vi "SysExe.Test Async StdIn and StdOut.vi"() -> ()   [LabVIEW 2018]
panel:
  in  "App":path=path "cmd.exe"
  out "Error":errorcluster
  out "Write StdIn":errorcluster
  out "StdOut":string
  in  "StdIn":string
  in  "stop":bool
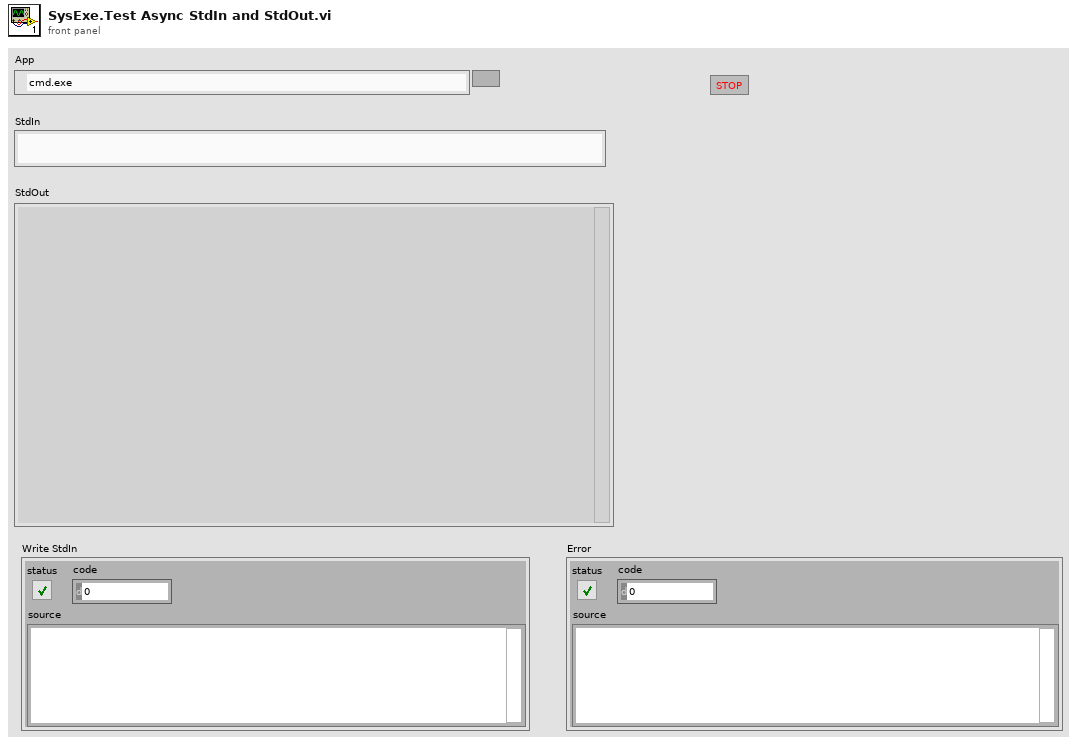
[diagram p1: front panel]
types:
  T1 = cluster{"Process":refnum<k24>, "StdIn":refnum<k24>, "StdErr":refnum<k24>, "StdOut":refnum<k24>, "StdOutDat":string, "StdErrDat":string, "StdInDat":string, "Args":string, "App":string, "AppFolder":path, "WorkingFolder":path, "IsRunning":bool, "Error":errorcluster, "StdOutCallback":refnum<k27>}
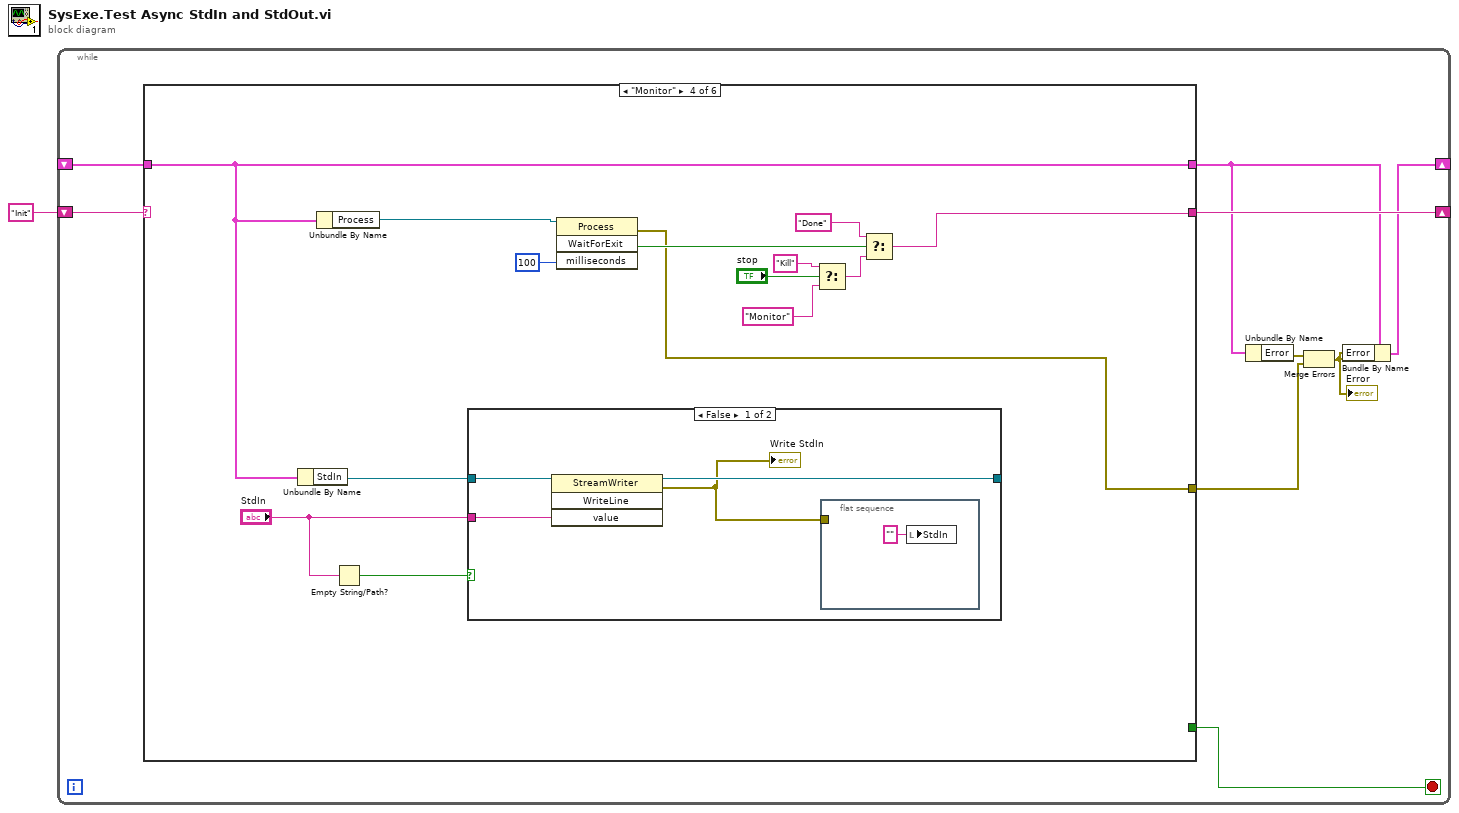
[diagram p0: block diagram]
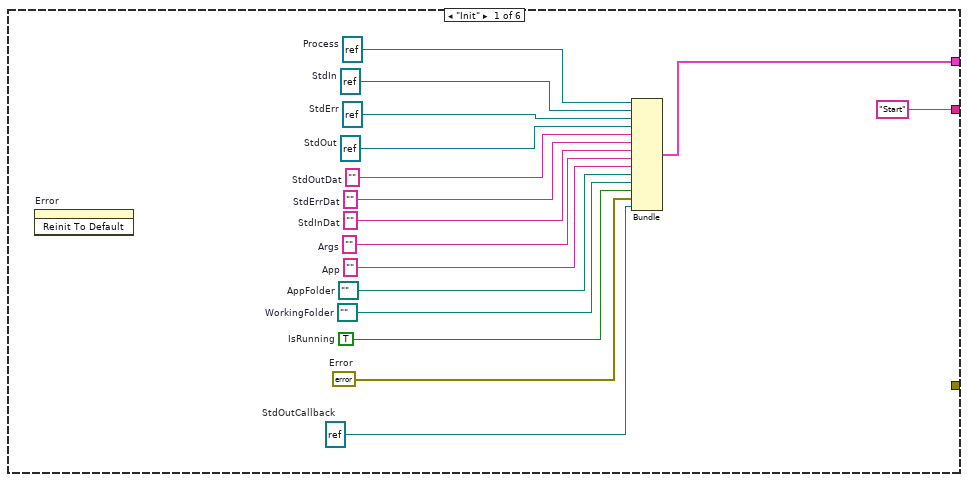
[diagram p2: hidden frame]
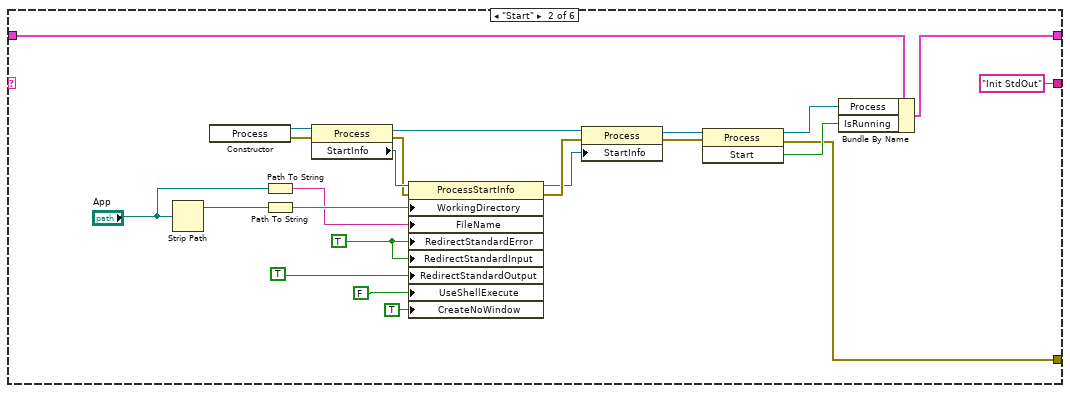
[diagram p3: hidden frame]
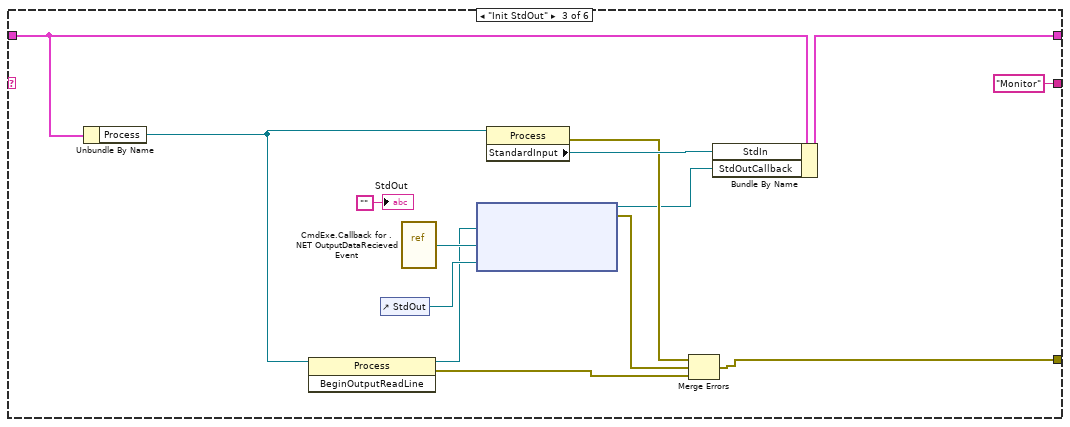
[diagram p4: hidden frame]
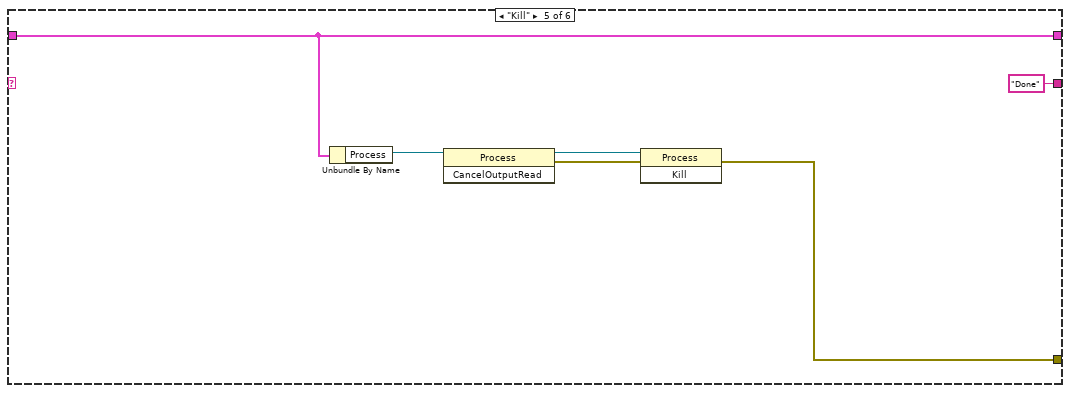
[diagram p6: hidden frame]
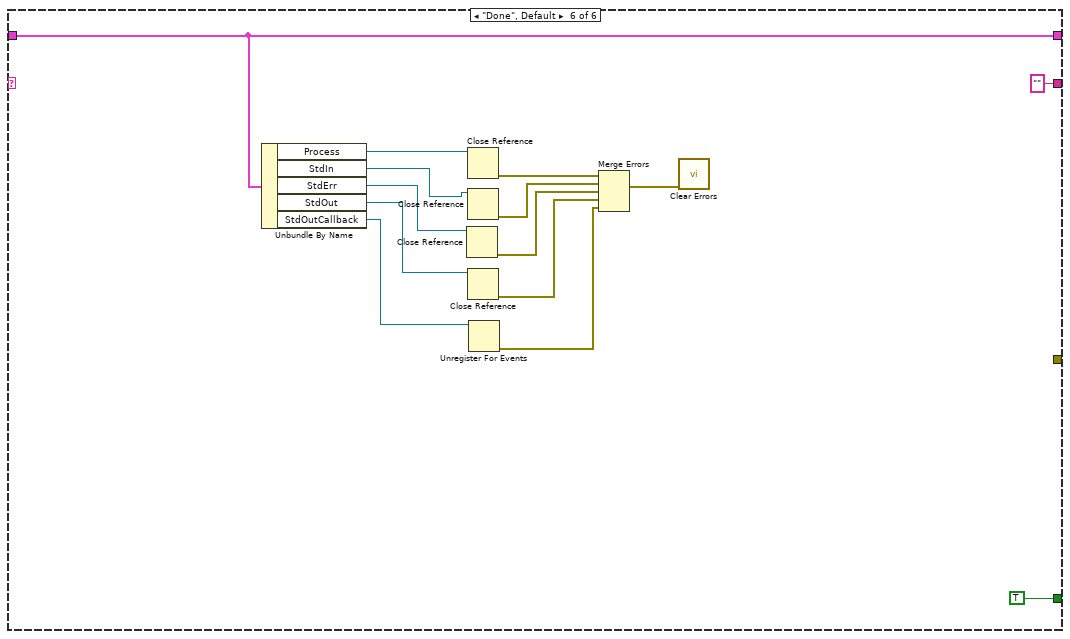
[diagram p7: hidden frame]
diagram:
  n1 = while {
    shift-right: [w6] -> _
    shift-left: _ -> [w8]
    shift-right: [w9] -> _
    shift-left: "Init" -> [w10]
    stop <- w7 stop-if-true
    n2 = case shown="\"Monitor\"" w10 {
      tunnel: [w18 w34 w56 w75 w88 w101] -> w5
      tunnel: ["Start" "Init StdOut" "Monitor" w67 "Done" "" ("StdIn")] -> w9
      tunnel: w8 -> [_ w35 w57 w75 w88 w101]
      tunnel: [_ _ _ _ _ TRUE] -> w7
      tunnel: [_ w31 w53 w66 w87 _] -> w2
      frame "Init" {
        w11 = refnum<k27> refnum  # StdOutCallback
        w12 = errorcluster {"status"=FALSE, "code"=0, "source"=""}  # Error
        w15 = TRUE  # IsRunning
        w16 = path ""  # WorkingFolder
        w17 = path ""  # AppFolder
        w13 = ""  # App
        w19 = ""  # Args
        w20 = ""  # StdInDat
        w21 = ""  # StdErrDat
        w22 = ""  # StdOutDat
        w23 = refnum<k24> refnum  # StdOut
        w24 = refnum<k24> refnum  # StdErr
        w25 = refnum<k24> refnum  # StdIn
        w26 = refnum<k24> refnum  # Process
        n3 = invoke on="Error" class="Clust (strict)" method="Reinit To Default"() -> ()  [unwired: 3 in, 3 out]
        n4 = Bundle("Process"=w26, "StdIn"=w25, "StdErr"=w24, "StdOut"=w23, "StdOutDat"=w22, "StdErrDat"=w21, "StdInDat"=w20, "Args"=w19, "App"=w13, "AppFolder"=w17, "WorkingFolder"=w16, "IsRunning"=w15, "Error"=w12, "StdOutCallback"=w11) -> (w18:T1)  [unwired: 1 in]
      }
      frame "Start" {
        w36 = TRUE ("UseShellExecute")
        n5 = Strip Path(path="App") -> (stripped path=w30:path)  [unwired: 1 out]
        n6 = constructor class="Process"() -> (reference out=w48:refnum<k24>, error out=w47:errorcluster)  [unwired: 3 in, 1 out]
        n7 = Path To String(path="App") -> (string=w27:string)
        n8 = Path To String(path=w30) -> (string=w29:string)
        n9 = property class="Process"(reference=w48, error in=w47) -> (reference out=w40:refnum<k24>, error out=w41:errorcluster, "StartInfo"=w46:refnum<k24>)
        n10 = property class="ProcessStartInfo"(reference=w46, error in=w41, "WorkingDirectory"=w29, "FileName"=w27, "RedirectStandardError"=w36, "RedirectStandardInput"=w36, "RedirectStandardOutput"=TRUE, "UseShellExecute"=FALSE, "CreateNoWindow"=TRUE) -> (reference out=w42:refnum<k24>, error out=w43:errorcluster)
        n11 = property class="Process"(reference=w40, error in=w43, "StartInfo"=w42) -> (reference out=w39:refnum<k24>, error out=w38:errorcluster)
        n12 = invoke class="Process" method="Start"(reference=w39, error in=w38) -> (reference out=w33:refnum<k24>, error out=w31:errorcluster, "Start"=w32:bool)  [unwired: 1 in]
        n13 = Bundle By Name(cluster=w35, "Process"=w33, "IsRunning"=w32) -> (w34:T1)
      }
      frame "Init StdOut" {
        n14 = Unbundle By Name(w57) -> ("Process"=w58:refnum<k24>)
        n15 = invoke class="Process" method="BeginOutputReadLine"(reference=w58) -> (reference out=w60:refnum<k24>, error out=w51:errorcluster)  [unwired: 2 in, 1 out]
        n16 = control-ref of="StdOut"() -> (w62:refnum<vi>)
        n17 = vi-ref "CmdExe.Callback for .NET OutputDataRecieved Event.vi"() -> ("vi reference"=w61:refnum<vi>)
        n18 = node(w60, w61, w62) -> (w50:refnum<k27>, w52:errorcluster)  [unwired: 2 in]
        n19 = property class="Process"(reference=w58) -> (error out=w54:errorcluster, "StandardInput"=w55:refnum<k24>)  [unwired: 1 in, 1 out]
        n20 = Merge Errors(w54, w52, w51) -> (w53:errorcluster)
        n21 = Bundle By Name(cluster=w57, "StdIn"=w55, "StdOutCallback"=w50) -> (w56:T1)
        "StdOut" <- ""
      }
      frame "Monitor" {
        n22 = Unbundle By Name(w75) -> ("StdIn"=w76:refnum<k24>)
        n23 = Unbundle By Name(w75) -> ("Process"=w74:refnum<k24>)
        n24 = Empty String/Path?(string/path="StdIn") -> (empty?=w64:bool)
        n25 = case shown="False" w64 {
          tunnel: w76 -> [w81 w83]
          tunnel: [w80 w83] -> _
          tunnel: "StdIn" -> [w78 _]
          frame False {
            n26 = invoke class="StreamWriter" method="WriteLine"(reference=w81, "value"=w78) -> (reference out=w80:refnum<k24>, error out=w79:errorcluster)  [unwired: 2 in, 2 out]
            "Write StdIn" <- w79
            n27 = flat-sequence {
              tunnel: w79 -> [_]
              frame #0 {
                n28 = local write "StdIn"("" ("StdIn")) -> ()
              }
            }
          }
          frame True {
          }
        }
        n29 = invoke class="Process" method="WaitForExit"(reference=w74, "milliseconds"=100) -> (error out=w66:errorcluster, "WaitForExit"=w73:bool)  [unwired: 2 in, 2 out]
        n30 = Select(t="Kill" ("StdIn"), s="stop", f="Monitor" ("StdIn")) -> (s? t:f=w71:string)
        n31 = Select(t="Done" ("StdIn"), s=w73, f=w71) -> (s? t:f=w67:string)
      }
      frame "Kill" {
        n32 = Unbundle By Name(w88) -> ("Process"=w86:refnum<k24>)
        n33 = invoke class="Process" method="CancelOutputRead"(reference=w86) -> (reference out=w85:refnum<k24>, error out=w84:errorcluster)  [unwired: 2 in, 1 out]
        n34 = invoke class="Process" method="Kill"(reference=w85, error in=w84) -> (error out=w87:errorcluster)  [unwired: 1 in, 2 out]
      }
      frame "Done", Default {
        n35 = Unbundle By Name(w101) -> ("Process"=w100:refnum<k24>, "StdIn"=w99:refnum<k24>, "StdErr"=w98:refnum<k24>, "StdOut"=w97:refnum<k24>, "StdOutCallback"=w91:refnum<k27>)
        n36 = Close Reference(reference=w98) -> (error out=w94:errorcluster)  [unwired: 1 in]
        n37 = Close Reference(reference=w100) -> (error out=w96:errorcluster)  [unwired: 1 in]
        n38 = Close Reference(reference=w99) -> (error out=w95:errorcluster)  [unwired: 1 in]
        n39 = Close Reference(reference=w97) -> (error out=w93:errorcluster)  [unwired: 1 in]
        n40 = Unregister For Events(event registration refnum=w91) -> (error out=w90:errorcluster)  [unwired: 1 in]
        n41 = Merge Errors(w96, w95, w94, w93, w90) -> (w92:errorcluster)
        n42 = call <vilib>:"Clear Errors.vi"("error in (no error)"=w92) -> ()  [unwired: 5 in, 2 out]
      }
    }
    n43 = Unbundle By Name(w5) -> ("Error"=w4:errorcluster)
    n44 = Merge Errors(w4, w2) -> (w3:errorcluster)
    "Error" <- w3
    n45 = Bundle By Name(cluster=w5, "Error"=w3) -> (w6:T1)
  }
